vi "AIT 1553 - Create BC Sysdef Tree Messages.vi"(7 "Called From SysDef API (F)":bool, 8 "error in":errorcluster, 9 "BC Messages":T1[](array[typedef]), 10 "Section Ptr":T3 format="%.0x") -> (0 "error out":errorcluster)   [LabVIEW 2013, in "AIT 1553 Custom Device.lvlib"]
uses:
  AIT 1553 Custom Device.lvlib
  <vilib>/NI Veristand/Custom Device API/Custom Device Item Ref.ctl
  Controls/1553_BC_Message.ctl
  Controls/1553 Param.ctl
  <vilib>/NI Veristand/Custom Device API/Custom Device Channel Type.ctl
  <vilib>/NI Veristand/Custom Device API/Custom Device Channel.ctl
  Controls and Global/Global.vi
  <vilib>/NI Veristand/Custom Device API/Custom Device API.lvlib
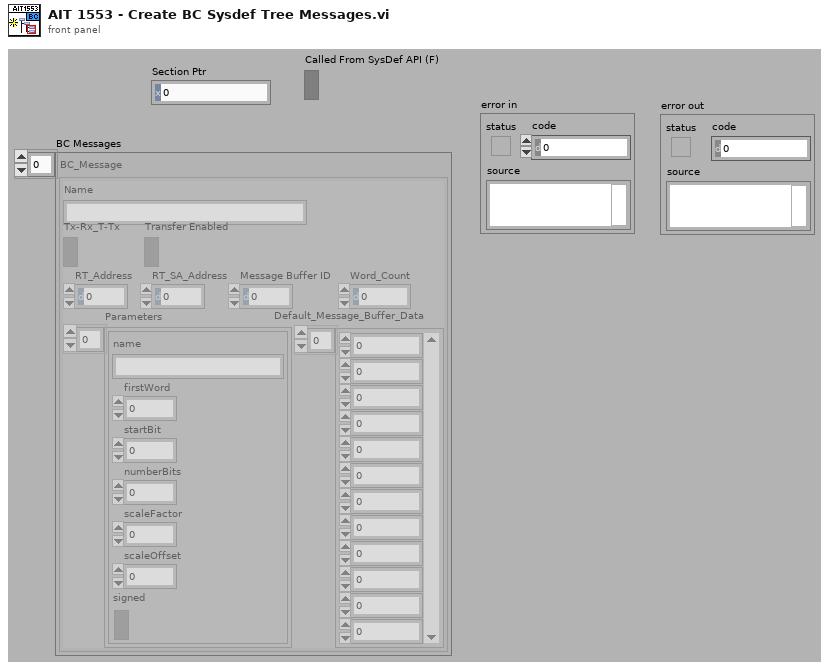
[diagram p1: front panel]
types:
  T1 = typedef "AIT 1553 Custom Device.lvlib/1553_BC_Message.ctl" = cluster{"Name":string, "Tx-Rx_T-Tx":bool, "RT_Address":u8, "RT_SA_Address":u8, "Parameters":T2[], "Transfer Enabled":bool, "Message Buffer ID":u16, "Default_Message_Buffer_Data":u16[], "Word_Count":u8}
  T2 = typedef "AIT 1553 Custom Device.lvlib/1553 Param.ctl" = cluster{"name":string, "firstWord":i32, "startBit":i32, "numberBits":i32, "scaleFactor":dbl, "scaleOffset":dbl, "signed":bool}
  T3 = typedef "Custom Device API.lvlib/Custom Device Item Ref.ctl" = u64
  T4 = typedef "Custom Device API.lvlib/Custom Device Channel.ctl" = cluster{"Type":T5, "Units":string, "Default Value":dbl, "Faultable":bool, "Scalable":bool}
  T5 = typedef "Custom Device API.lvlib/Custom Device Channel Type.ctl" = enum16{"Input", "Output"}
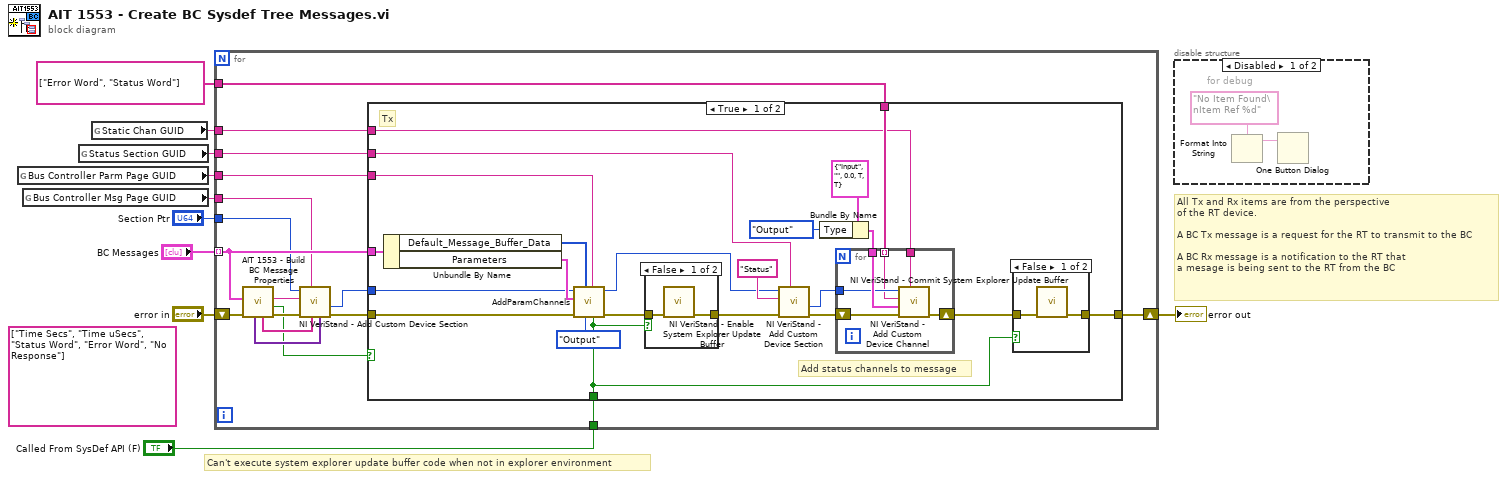
[diagram p0: block diagram]
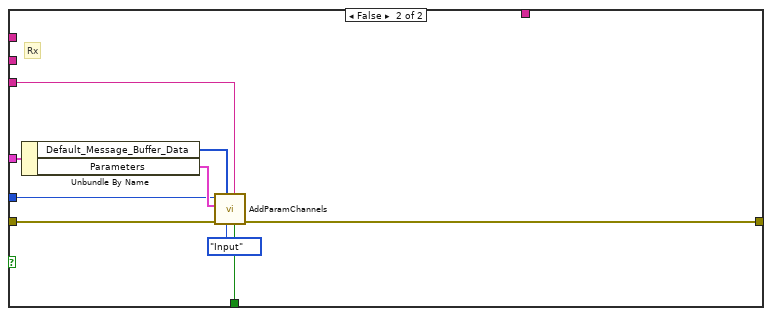
[diagram p5: hidden frame]
diagram:
  (unwired) string[] ["Time Secs", "Time uSecs", "Status Word", "Error Word", "No Response"]
  # "Can't execute system explorer update buffer code when not in explorer environment"
  # "All Tx and Rx items are from the perspective \nof the RT device.\n\nA BC Tx message is a request for the RT to transmit to the BC\n\nA BC Rx message is a notification to the RT that\na mesage is being sent to the RT from the BC"
  n1 = global read "Global.vi" "Bus Controller Parm Page GUID"() -> (w4:string)
  n2 = global read "Global.vi" "Bus Controller Msg Page GUID"() -> (w7:string)
  n3 = global read "Global.vi" "Status Section GUID"() -> (w2:string)
  n4 = global read "Global.vi" "Static Chan GUID"() -> (w6:string)
  n5 = for {
    shift-right: [w12] -> w10
    shift-left: "error in" -> [w23]
    tunnel: "Section Ptr" -> [w20]
    tunnel: "BC Messages" -> [w22] mode=indexing
    tunnel: w7 -> [w21]
    tunnel: w6 -> [w13]
    tunnel: w4 -> [w19]
    tunnel: string[] ["Error Word", "Status Word"] -> [w14]
    tunnel: w2 -> [w15]
    tunnel: "Called From SysDef API (F)" -> [w11]
    n6 = call "AIT 1553 - Build BC Message Properties.vi"("error in (no error)"=w23, "BC_Message"=w22) -> ("error out"=w25:errorcluster, "Tx-Rx  (T=Tx)"=w16:bool, "name"=w24:string, "Prop Names"=w26:string[], "Prop Values"=w27:variant[])  [unwired: 5 in]
    n7 = call <vilib>:"NI VeriStand - Add Custom Device Section.vi"("Property Values"=w27, "Property names"=w26, "GUID (Default Section)"=w21, "error in (no error)"=w25, "Section Name"=w24, "Parent Ref in"=w20) -> ("error out"=w18:errorcluster, "Section Ptr"=w17:T3)  [unwired: 2 in, 2 out]
    n8 = case shown="True" w16 {
      tunnel: w18 -> [w48 w69]
      tunnel: w17 -> [w47 w68]
      tunnel: [w34 w65] -> w12
      tunnel: w22 -> [w45 w66]
      tunnel: w19 -> [w43 w63]
      tunnel: w15 -> [w33 _]
      tunnel: w14 -> [w32 _]
      tunnel: w13 -> [w31 _]
      tunnel: w11 -> [w29 w62]
      frame True {
        # "Add status channels to message"
        # "Tx"
        n9 = Unbundle By Name(w45) -> ("Default_Message_Buffer_Data"=w44:u16[], "Parameters"=w49:T2[])
        n10 = call "AddParamChannels.vi"("Called From SysDef API (F)"=w29, "Parm Page GUID"=w43, "Type"=Custom_Device_Channel_Type."Output", "Default Message Data"=w44, "error in"=w48, "Parameters to add"=w49, "Node Ref In"=w47) -> ("error out"=w35:errorcluster, "Node Ref Out"=w30:T3)  [unwired: 3 in]
        n11 = case shown="False" w29 {
          tunnel: [w54 w55] -> w42
          tunnel: w35 -> [w53 w55]
          frame False {
            n12 = call <vilib>:"NI VeriStand - Enable System Explorer Update Buffer.vi"("error in (no error)"=w53) -> ("error out"=w54:errorcluster)  [unwired: 10 in]
          }
          frame True {
          }
        }
        n13 = call <vilib>:"NI VeriStand - Add Custom Device Section.vi"("GUID (Default Section)"=w33, "error in (no error)"=w42, "Section Name"="Status", "Parent Ref in"=w30) -> ("error out"=w39:errorcluster, "Section Ptr"=w40:T3)  [unwired: 4 in, 2 out]
        n14 = Bundle By Name(cluster=T4 {"Type"=enum."Input", "Units"="", "Default Value"=0.0, "Faultable"=TRUE, "Scalable"=TRUE} ("Channel"), "Type"=Custom_Device_Channel_Type."Output") -> (w38:T4)
        n15 = for {
          tunnel: w38 -> [w60]
          tunnel: w31 -> [w59]
          tunnel: w40 -> [w57]
          tunnel: w32 -> [w56] mode=indexing
          shift-right: [w61] -> w28
          shift-left: w39 -> [w58]
          n16 = call <vilib>:"NI VeriStand - Add Custom Device Channel.vi"("GUID (Default Channel)"=w59, "error in (no error)"=w58, "Channel"=w60, "Channel Name"=w56, "Parent Ref in"=w57) -> ("error out"=w61:errorcluster)  [unwired: 3 in, 3 out]
        }
        n17 = case shown="False" w29 {
          tunnel: w28 -> [w51 w52]
          tunnel: [w50 w52] -> w34
          frame False {
            n18 = call <vilib>:"NI VeriStand - Commit System Explorer Update Buffer.vi"("error in (no error)"=w51) -> ("error out"=w50:errorcluster)  [unwired: 10 in]
          }
          frame True {
          }
        }
      }
      frame False {
        # "Rx"
        n19 = Unbundle By Name(w66) -> ("Default_Message_Buffer_Data"=w64:u16[], "Parameters"=w70:T2[])
        n20 = call "AddParamChannels.vi"("Called From SysDef API (F)"=w62, "Parm Page GUID"=w63, "Type"=Custom_Device_Channel_Type."Input", "Default Message Data"=w64, "error in"=w69, "Parameters to add"=w70, "Node Ref In"=w68) -> ("error out"=w65:errorcluster)  [unwired: 3 in, 1 out]
      }
    }
  }
  "error out" <- w10
  n21 = disable-structure shown="Disabled" {
    frame Disabled {
      # "for debug"
      n22 = Format Into String(format string="No Item Found\nItem Ref %d" ("message")) -> (resulting string=w73:string, w71:T3)  [unwired: 2 in, 1 out]
      n23 = One Button Dialog(message=w73) -> (true=w74:bool)  [unwired: 1 in]
    }
    frame Enabled {
    }
  }
